vi "Example - Main.vi"() -> ()   [LabVIEW 2015]
uses:
  lvlib/LV-Proof-Reading.lvlib
panel:
  in  "Process":bool
  in  "Suggestion":i32(listbox)
  in  "Input Text":string
  in  "Application ID":string
  # "Web Services by Yahoo! JAPAN ( https://developer.yahoo.co.jp/sitemap/)"
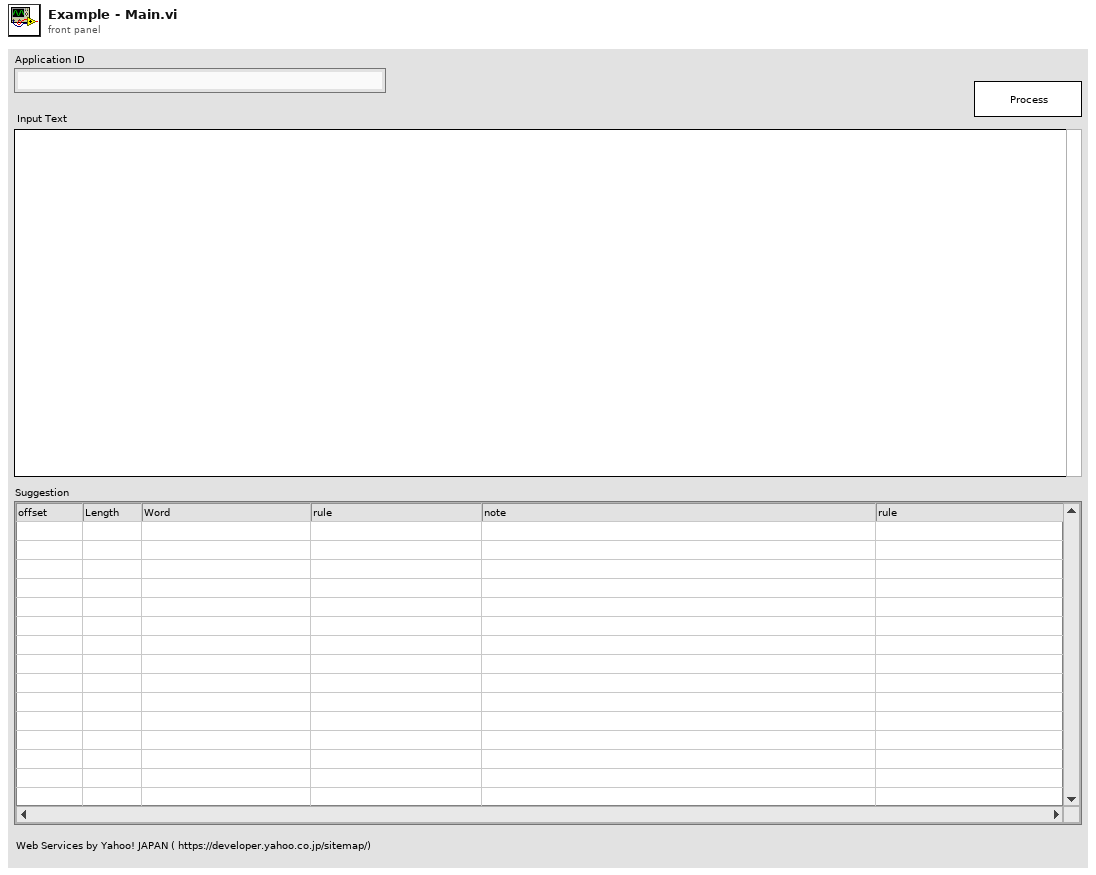
[diagram p1: front panel]
types:
  T1 = typedef "LV-Proof-Reading.lvlib/suggestion.ctl" = cluster{"offset":i32, "length":i32, "note":string, "rule":string, "suggestion":string, "word":string}
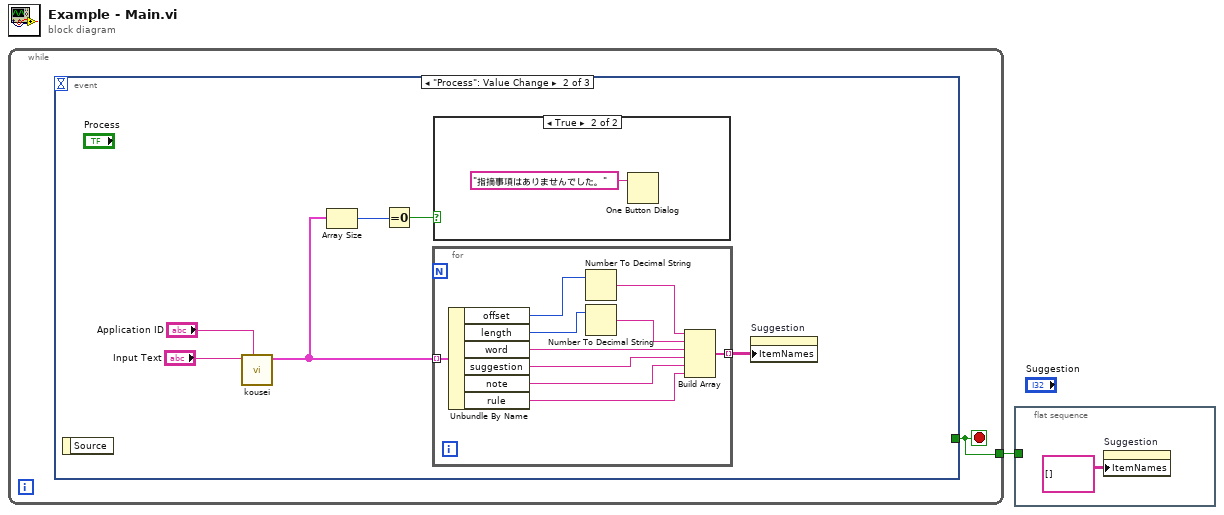
[diagram p0: block diagram]
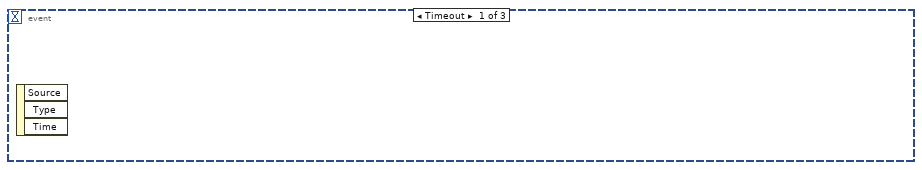
[diagram p2: hidden frame]
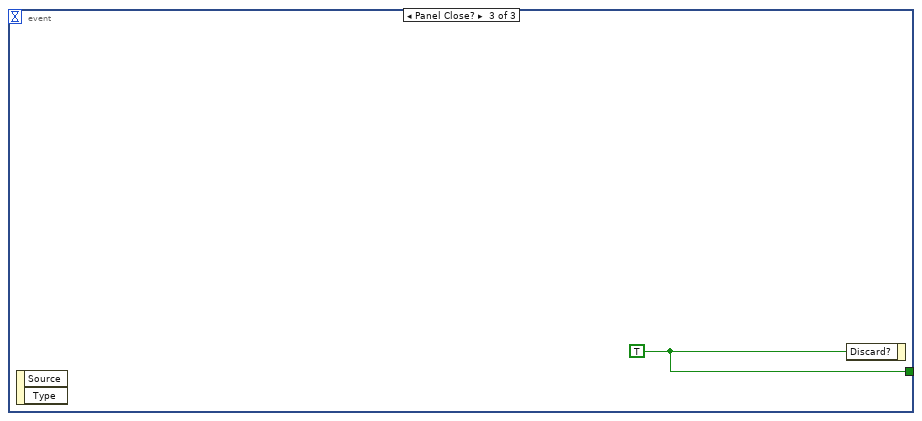
[diagram p4: hidden frame]
diagram:
  n1 = while {
    tunnel: [w2] -> w1
    stop <- w2 stop-if-true
    n2 = event shown="[1] \"Process\": Value Change" {
      selector: _ -> [_ _ _]
      dyn-events: _ -> [_ _ _]
      timeout: _ -> [_ _ _]
      tunnel: [_ _ w20] -> w2
      event Timeout {
        n3 = event-data() -> ()  [unwired: 1 in, 3 out]
      }
      event "Process": Value Change {
        n4 = event-data() -> ()  [unwired: 1 in, 1 out]
        n5 = call "kousei.vi"("Application ID"="Application ID", "Input Text"="Input Text") -> ("Suggestion"=w5:T1[])  [unwired: 8 in, 1 out]
        n6 = Array Size(array=w5) -> (size(s)=w4:i32)
        n7 = Equal To 0?(x=w4) -> (x = 0?=w3:bool)
        n8 = for {
          tunnel: w5 -> [w19] mode=indexing
          tunnel: [w13] -> w8 mode=indexing
          n9 = Unbundle By Name(w19) -> ("offset"=w18:i32, "length"=w17:i32, "word"=w14:string, "suggestion"=w10:string, "note"=w12:string, "rule"=w11:string)
          n10 = Number To Decimal String(number=w18) -> (decimal integer string=w16:string)  [unwired: 1 in]
          n11 = Number To Decimal String(number=w17) -> (decimal integer string=w15:string)  [unwired: 1 in]
          n12 = Build Array(w16, w15, w14, w10, w12, w11) -> (w13:string[])
        }
        n13 = case shown="True" w3 {
          frame False {
          }
          frame True {
            n14 = One Button Dialog(message="指摘事項はありませんでした。") -> ()  [unwired: 1 in, 1 out]
          }
        }
        n15 = property on="Suggestion" class="MCListbox (strict)"("ItemNames"=w8) -> ()  [unwired: 2 in, 2 out]
      }
      event Panel Close? {
        w20 = TRUE ("Discard?")
        n16 = event-data() -> ()  [unwired: 1 in, 2 out]
        n17 = event-data("Discard?"=w20) -> ()  [unwired: 1 in, 1 out]
      }
    }
  }
  n18 = flat-sequence {
    tunnel: w1 -> [_]
    frame #0 {
      n19 = property on="Suggestion" class="MCListbox (strict)"("ItemNames"=string[][] [] ("Item Names")) -> ()  [unwired: 2 in, 2 out]
    }
  }
